vi "TAT-Read Reciepe.vi"(8 "error in (no error)":errorcluster) -> (0 "error out":errorcluster, 2 "Part Name":string, 3 "Data To Load":T1 {"T-Bin Seq. Select"."First" max=8 step=1; "T-Bin Seq. Select"."Second" max=8 step=1; "T-Bin Seq. Select"."Third" max=8 step=1; "T-Bin Seq. Select"."Fourth" max=8 step=1; "T-Bin Seq. Select"."Fifth" max=8 step=1; "T-Bin Seq. Select"."Sixth" max=8; "Ass. Sensor Select"."Gun \nProg No." max=8 step=1; "Ass. Sensor Select"."Camera-2 \nProg No." max=8 step=1; "Ass. Sensor Select"."Camera-1 \nProg No." max=8 step=1})   [LabVIEW 2017]
uses:
  Controls/Recipe.ctl
  <vilib>/Utility/config.llb/Read Key (String).vi
  <vilib>/Utility/config.llb/NI_LVConfig.lvlib
panel:
  in  "LOAD":bool
  in  "PART NAME":string(combo)
  # "SELECT RECIEPE"
  # "Bin No."
  # "Bin No."
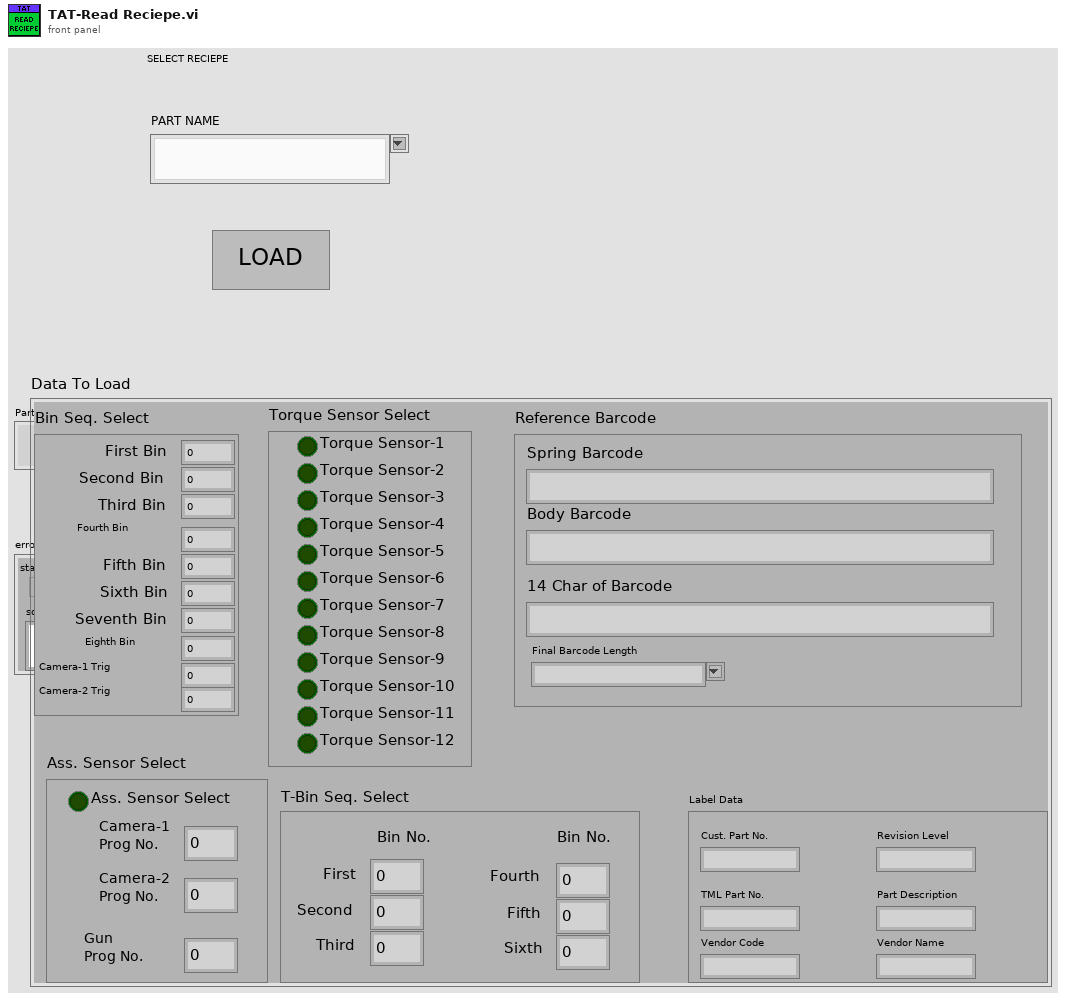
[diagram p1: front panel]
types:
  T1 = typedef "Recipe.ctl" = cluster{"Ass. Sensor Select":cluster{"Ass. Sensor Select":bool, "Camera-1 \nProg No.":u16, "Camera-2 \nProg No.":u16, "Gun \nProg No.":u16}, "Torque Sensor Select":cluster{"Torque Sensor-1":bool, "Torque Sensor-2":bool, "Torque Sensor-3":bool, "Torque Sensor-4":bool, "Torque Sensor-5":bool, "Torque Sensor-6":bool, "Torque Sensor-7":bool, "Torque Sensor-8":bool, "Torque Sensor-9":bool, "Torque Sensor-10":bool, "Torque Sensor-11":bool, "Torque Sensor-12":bool}, "Bin Seq. Select":cluster{"First Bin":u16, "Second Bin":u16, "Third Bin":u16, "Fourth Bin":u16, "Fifth Bin":u16, "Sixth Bin":u16, "Seventh Bin":u16, "Eighth Bin":u16, "Camera-1 Trig":u16, "Camera-2 Trig":u16}, "T-Bin Seq. Select":cluster{"First":u16, "Second":u16, "Third":u16, "Fourth":u16, "Fifth":u16, "Sixth":u16}, "Reference Barcode":cluster{"Spring Barcode":string, "Body Barcode":string, "14 Char of Barcode":string, "Final Barcode Length":string}, "Label Data":cluster{"Cust. Part No.":string, "TML Part No.":string, "Vendor Code":string, "Revision Level":string, "Part Description":string, "Vendor Name":string}}
  T2 = enum32{"invalid app kind", "Development System", "Run Time System", "Student Edition", "Embedded LabVIEW", "Evaluation", "Custom"}
  T3 = typedef "NI_LVConfig.lvlib/Config Data RefNum.ctl" = refnum<k1>
  T4 = enum32{"Invalid", "Standard", "Closed", "Hidden", "Minimized", "Maximized"}
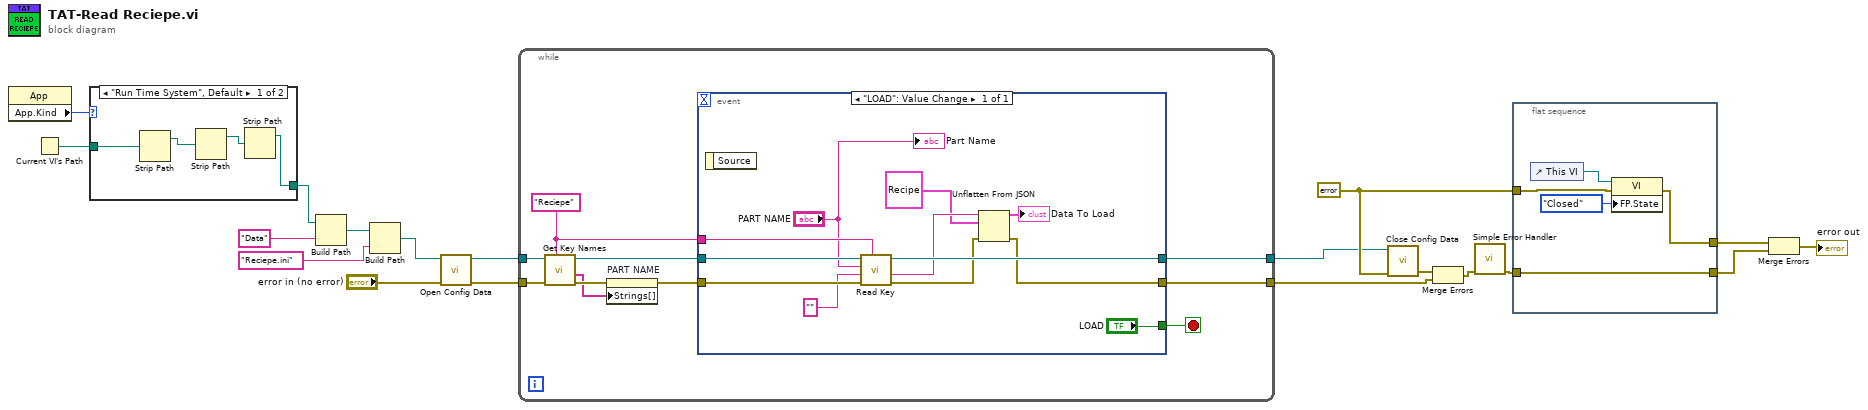
[diagram p0: block diagram]
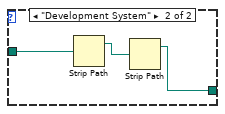
[diagram p2: hidden frame]
diagram:
  w8 = errorcluster {"status"=FALSE, "code"=0, "source"=""} ("error in (no error)")
  n1 = property class="App"() -> ("App.Kind"=w18:T2)  [unwired: 2 in, 2 out]
  n2 = Current VI's Path() -> (path=w19:path)
  n3 = case shown="\"Run Time System\", Default" w18 {
    tunnel: w19 -> [w21 w25]
    tunnel: [w20 w24] -> w16
    frame "Run Time System", Default {
      n4 = Strip Path(path=w21) -> (stripped path=w23:path)  [unwired: 1 out]
      n5 = Strip Path(path=w23) -> (stripped path=w22:path)  [unwired: 1 out]
      n6 = Strip Path(path=w22) -> (stripped path=w20:path)  [unwired: 1 out]
    }
    frame "Development System" {
      n7 = Strip Path(path=w25) -> (stripped path=w26:path)  [unwired: 1 out]
      n8 = Strip Path(path=w26) -> (stripped path=w24:path)  [unwired: 1 out]
    }
  }
  n9 = Build Path(base path=w16, name or relative path="Data") -> (appended path=w17:path)
  n10 = Build Path(base path=w17, name or relative path="Reciepe.ini") -> (appended path=w15:path)
  n11 = call <vilib>:"Open Config Data.vi"("error in (no error)"="error in (no error)", "configuration file path"=w15) -> ("error out"=w5:errorcluster, "refnum"=w3:T3)  [unwired: 7 in, 1 out]
  n12 = while {
    tunnel: [w35] -> w6
    tunnel: w5 -> [w33]
    tunnel: [w34] -> w4
    tunnel: w3 -> [w32]
    stop <- w36 stop-if-true
    w30 = "Reciepe" ("section")
    n13 = call <vilib>:"Get Key Names.vi"("section"=w30, "error in (no error)"=w33, "refnum"=w32) -> ("error out"=w29:errorcluster, "key names"=w27:string[], "refnum out"=w31:T3)  [unwired: 5 in, 1 out]
    n14 = property on="PART NAME" class="CmbBox"(error in=w29, "Strings[]"=w27) -> (error out=w28:errorcluster)  [unwired: 1 in, 1 out]
    n15 = event shown="[0] \"LOAD\": Value Change" {
      selector: _ -> [_]
      dyn-events: _ -> [_]
      timeout: _ -> [_]
      tunnel: ["LOAD"] -> w36
      tunnel: [w41] -> w35
      tunnel: w28 -> [w45]
      tunnel: [w46] -> w34
      tunnel: w31 -> [w47]
      tunnel: w30 -> [w40]
      event "LOAD": Value Change {
        n16 = event-data() -> ()  [unwired: 1 in, 1 out]
        n17 = call-poly <vilib>:"Read Key.vi"("section"=w40, "error in (no error)"=w45, "default value"="", "key"="PART NAME", "refnum"=w47) -> ("error out"=w42:errorcluster, "value"=w43:string, "refnum out"=w46:T3)  [unwired: 3 in, 1 out]
        n18 = Unflatten From JSON(JSON string=w43, type and defaults=T1 {"Ass. Sensor Select"={"Ass. Sensor Select"=FALSE, "Camera-1 \nProg No."=0, "Camera-2 \nProg No."=0, "Gun \nProg No."=0}, "Torque Sensor Select"={"Torque Sensor-1"=FALSE, "Torque Sensor-2"=FALSE, "Torque Sensor-3"=FALSE, "Torque Sensor-4"=FALSE, "Torque Sensor-5"=FALSE, "Torque Sensor-6"=FALSE, "Torque Sensor-7"=FALSE, "Torque Sensor-8"=FALSE, "Torque Sensor-9"=FALSE, "Torque Sensor-10"=FALSE, "Torque Sensor-11"=FALSE, "Torque Sensor-12"=FALSE}, "Bin Seq. Select"={"First Bin"=0, "Second Bin"=0, "Third Bin"=0, "Fourth Bin"=0, "Fifth Bin"=0, "Sixth Bin"=0, "Seventh Bin"=0, "Eighth Bin"=0, "Camera-1 Trig"=0, "Camera-2 Trig"=0}, "T-Bin Seq. Select"={"First"=0, "Second"=0, "Third"=0, "Fourth"=0, "Fifth"=0, "Sixth"=0}, "Reference Barcode"={"Spring Barcode"="", "Body Barcode"="", "14 Char of Barcode"="", "Final Barcode Length"=""}, "Label Data"={"Cust. Part No."="", "TML Part No."="", "Vendor Code"="", "Revision Level"="", "Part Description"="", "Vendor Name"=""}}, error in (no error)=w42) -> (value=→"Data To Load":T1, error out=w41:errorcluster)  [unwired: 4 in]
        "Part Name" <- "PART NAME"
      }
    }
  }
  n19 = call <vilib>:"Close Config Data.vi"("error in (no error)"=w8, "refnum"=w4) -> ("error out"=w12:errorcluster)  [unwired: 8 in, 1 out]
  n20 = Merge Errors(w12, w6) -> (w7:errorcluster)
  n21 = call <vilib>:"Simple Error Handler.vi"("error in (no error)"=w7) -> ("error out"=w9:errorcluster)  [unwired: 4 in, 4 out]
  n22 = flat-sequence {
    tunnel: w8 -> [w51]
    tunnel: [w50] -> w11
    tunnel: [w49] -> w10
    tunnel: w9 -> [w49]
    frame #0 {
      n23 = control-ref of="This VI"() -> (w53:refnum<vi>)
      n24 = property class="VI"(reference=w53, error in=w51, "FP.State"=T4."Closed" ("Front Panel Window:State")) -> (error out=w50:errorcluster)  [unwired: 1 out]
    }
  }
  n25 = Merge Errors(w11, w10) -> (→"error out":errorcluster)
